vi "Status.Builder.Set State Pointer.vi"(10 "Builder State Pointer":refnum<class "DSF.Engine.Pointer.Status.Builder.State.lvclass">, 11 "Builder Status in":refnum<class "Status.Builder.lvclass">) -> (3 "Builder Status out":refnum<class "Status.Builder.lvclass">)   [LabVIEW 2017, in "DSF.Engine.lvlib" / "Status.Builder.lvclass"]
uses:
  Status.Builder.lvclass
  Pointer/DSF.Engine.Pointer.Status.Builder.State.lvclass
  Status.Builder.lvclass/Status.Builder.ctl
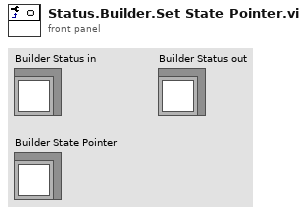
[diagram p1: front panel]
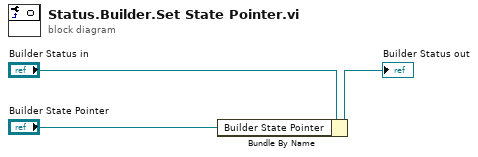
[diagram p0: block diagram]
diagram:
  n1 = Bundle By Name(cluster="Builder Status in", "Builder State Pointer"="Builder State Pointer") -> (→"Builder Status out":refnum<class "Status.Builder.lvclass">)
